vi "Kinesis - KDC101 - Motor Status Changed.vi"() -> ()   [LabVIEW 2017]
uses:
  U:/Kinesis LabVIEW Website Examples/Thorlabs.MotionControl.Controls.dll
  Thorlabs.MotionControl.Controls.dll
  U:/Kinesis LabVIEW Website Examples/ThorLabs.MotionControl.KCube.DCServoCLI.dll
  ThorLabs.MotionControl.KCube.DCServoCLI.dll
panel:
  in  "?":bool
  in  "SerialNumber":string
  in  "KCubeDCServoControl":refnum<k24>(container)
  # "Notes:"
  # "- Ensure that the appropriate .DLLs are copied into your Project Folder. Check that the correct bit type are used depending on your version of LabVIEW\ni.e. 32-bit or 64-bit.\n\n\n\n\n\n\n\n\n\n\n\n\n\n\n- Open the example VI through the LabVIEW Project Explorer to correctly load the User Interface from Thorlabs.MotionControl.Controls.dll."
  # "Thorlabs Hardware: KDC101 - K-Cube Brushed DC Servo Motor Controller\nhttps://www.thorlabs.com/newgrouppage9.cfm?objectgroup_id=2419\n\nDescription: This VI will enable you to make use of Motor Events. These events include Motor Status & Connection Change Events, Settings Update Events  as well as Error Update Events. In this instance we make use of the Motor Status update.\nAn Event Callback Sub-VI is accessed using the Register Event Callback Function in LabVIEW. When 'Run', the user will be prompted with a message when the Motor state changes from 'Idle' to 'Moving'.\n\nInstructions: \n1) Connect your KDC101 device to your PC & power the device, ensuring your stage/actutator is connected. For full device setup, the device product manual can be found on our website here. - https://www.thorlabs.com/thorproduct.cfm?partnumber=KDC101\n2) Enter the device serial number below.\n3) Click 'Run' in the LabVIEW Toolbar.\n4) To end the VI, click the 'END PROGRAM' button."
  # "Example Image of .NET Controller - VI opened via Project Explorer/ not opened via Project Explorer"
  # "VI Not Opened via Project Explorer"
  # "VI Opened via Project Explorer"
  # "- To explore the range of methods available, please visit the .NET API, included with your Kinesis software.\n\n- For tips on building your own VIs with Thorlabs Motion Control Hardware, please see our LabVIEW Guide here.\nhttps://www.thorlabs.com/newgrouppage9.cfm?objectgroup_id=10285"
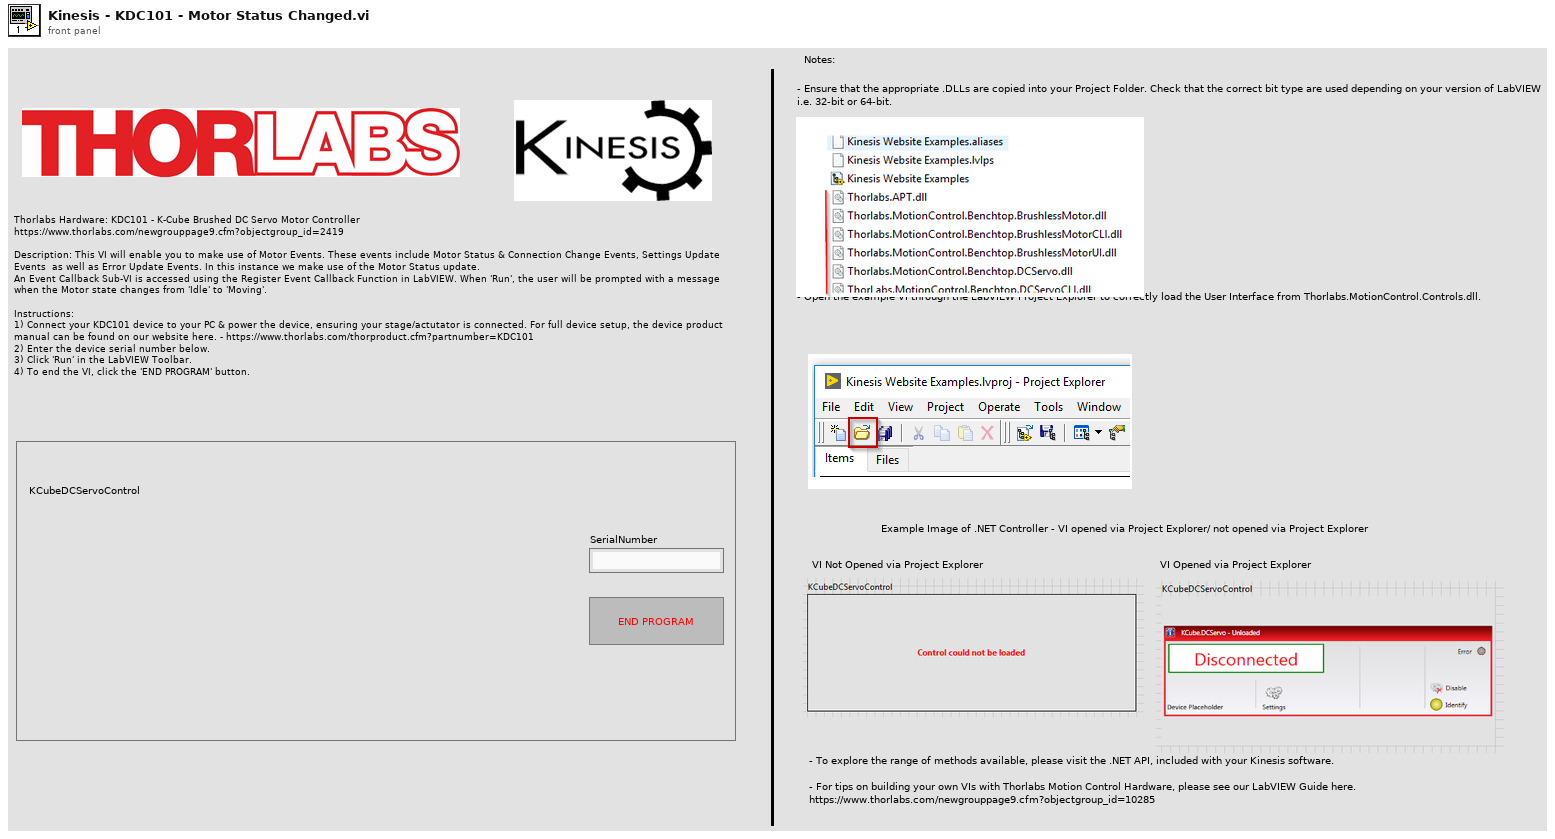
[diagram p1: front panel]
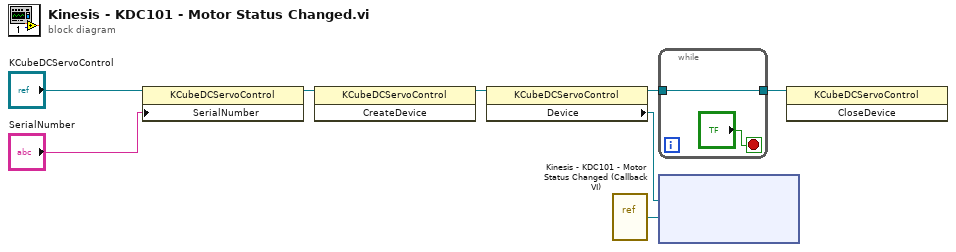
[diagram p0: block diagram]
diagram:
  n1 = property class="KCubeDCServoControl"(reference="KCubeDCServoControl", "SerialNumber"="SerialNumber") -> (reference out=w7:refnum<k24>)  [unwired: 1 in, 1 out]
  n2 = invoke class="KCubeDCServoControl" method="CreateDevice"(reference=w7) -> (reference out=w6:refnum<k24>)  [unwired: 2 in, 2 out]
  n3 = property class="KCubeDCServoControl"(reference=w6) -> (reference out=w1:refnum<k24>, "Device"=w4:refnum<k24>)  [unwired: 1 in, 1 out]
  n4 = vi-ref "Kinesis - KDC101 - Motor Status Changed (Callback VI).vi"() -> ("vi reference"=w3:refnum<vi>)
  n5 = while {
    tunnel: [w9] -> w2
    tunnel: w1 -> [w9]
    stop <- "?" stop-if-true
  }
  n6 = node(w4, w3) -> ()  [unwired: 3 in, 2 out]
  n7 = invoke class="KCubeDCServoControl" method="CloseDevice"(reference=w2) -> ()  [unwired: 2 in, 3 out]
